vi "Read Configuration.vi"(10 "XML File Path conf":path=path "c:/ni-rt/startup/configuration.xml", 11 "Error In":errorcluster) -> (0 "Matrices":T1, 1 "Configuration":T3={"Accelerometer Bias"={"X (m/s)"=0.0, "Y (m/s)"=0.0, "Z (m/s)"=0.0}, "Gyroscope Bias"={"X (m/s)"=0.0, "Y (m/s)"=0.0, "Z (m/s)"=0.0}, "Steering Motor Gear Ratio"=611.0, "Steering Pully Gear Ratio"=1.0, "Steering Encoder CPR"=500.0, "Steering Motor Max RPM"=4000.0, "Wheelbase (m)"=1.12, "Fork Angle (rad)"=1.3, "Balancing Controller"={"Kp (/s)"=0.0, "Kd (1)"=0.0}, "Max Allowed Steering Angle (rad)"=0.7, "Task Periods"={"Emergency Stop (us)"=0, "IMU (us)"=0, "Steering Motor Encoder (us)"=0, "State Estimator (us)"=0, "Balancing Controller (us)"=0, "GNSS (us)"=0, "Logging (us)"=0, "Drive Motor (us)"=0}, "Drive Motor Gear Ratio"=0.7, "Drive Motor UART Delay (ms)"=10}, 3 "Error Out":errorcluster)   [LabVIEW 2021]
uses:
  Configuration.ctl
  <vilib>/Analysis/Matrix/Datatypes/RealMatrix.ctl
  <vilib>/Utility/xml.llb/Read From XML File(string).vi
  <vilib>/Analysis/Matrix/Numeric/Conversions/Matrix To Array - RM.vi
  <vilib>/Analysis/Matrix/NI_Matrix.lvlib
panel:
  in  "init trajectory":dbl[][](array[numeric])
  in  "XML File Path traj":path=path "c:/ni-rt/startup/trajectorylab.xml"
  in  "Init Matrix":T2
  in  "XML File Path matr":path=path "c:/ni-rt/startup/matrixlab.xml"
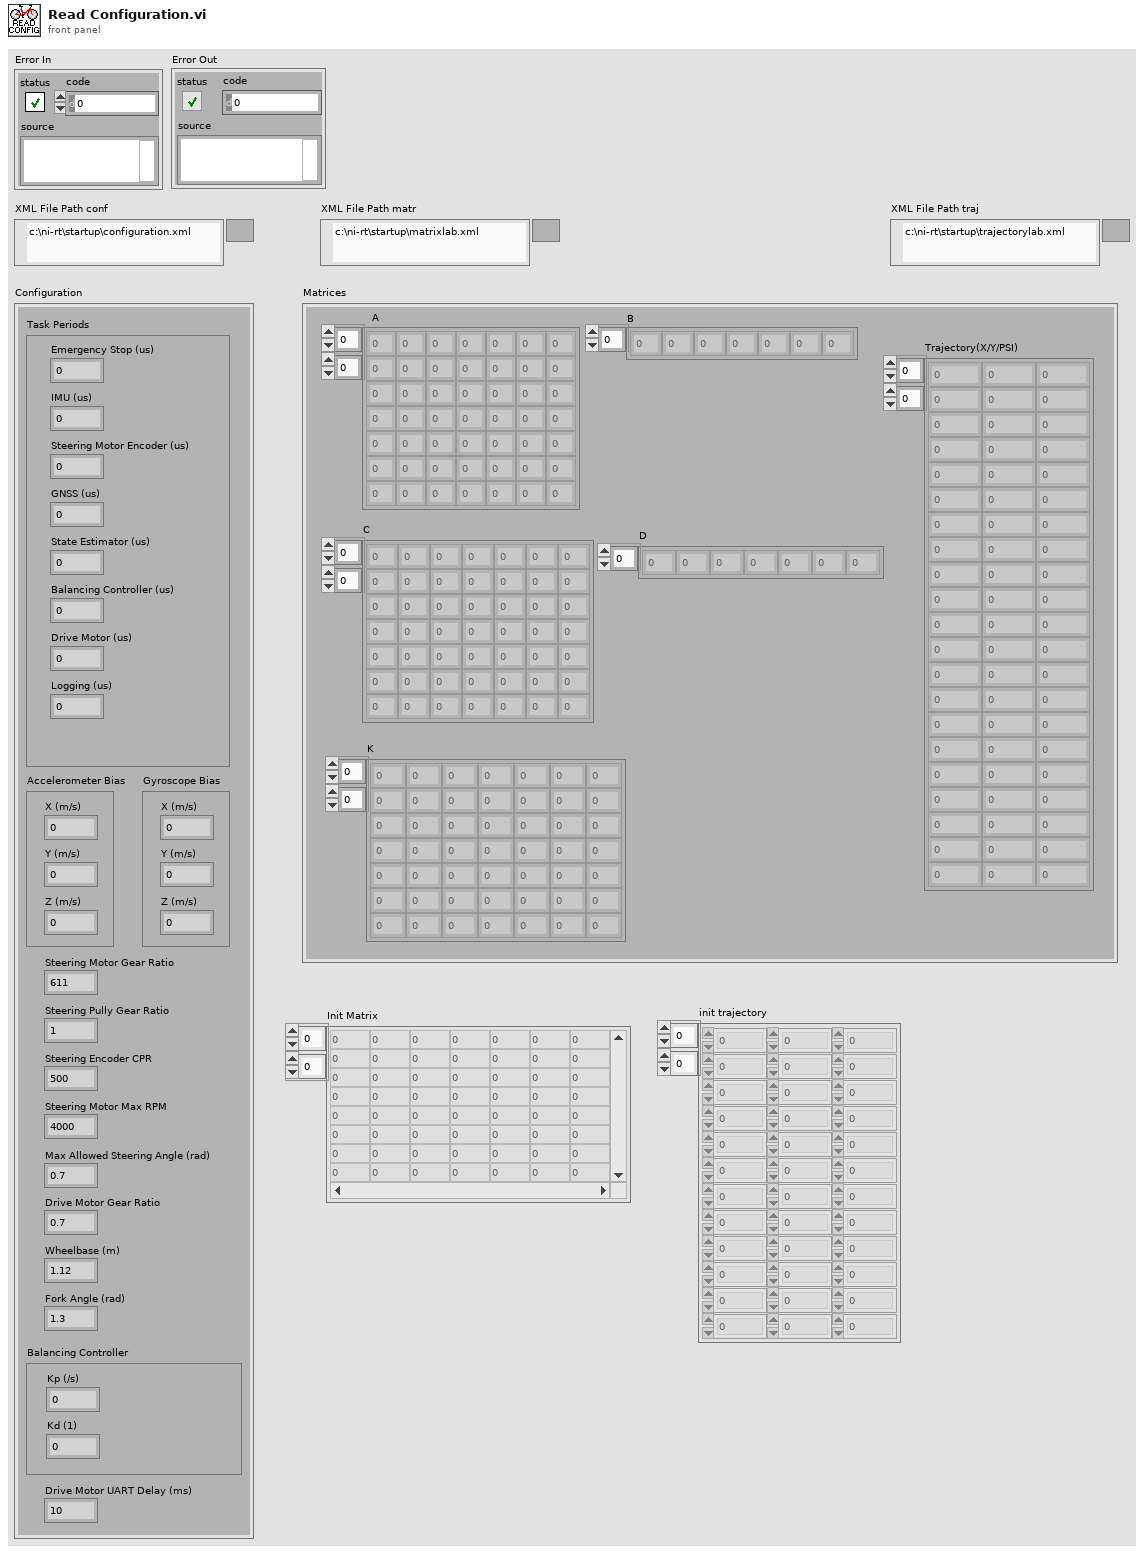
[diagram p1: front panel]
types:
  T1 = cluster{"B":dbl[], "A":dbl[][], "C":dbl[][], "D":dbl[], "K":dbl[][], "Trajectory(X/Y/PSI)":dbl[][]}
  T2 = typedef "NI_Matrix.lvlib/RealMatrix.ctl" = dbl[][]
  T3 = typedef "Configuration.ctl" = cluster{"Accelerometer Bias":cluster{"X (m/s)":dbl, "Y (m/s)":dbl, "Z (m/s)":dbl}, "Gyroscope Bias":cluster{"X (m/s)":dbl, "Y (m/s)":dbl, "Z (m/s)":dbl}, "Steering Motor Gear Ratio":dbl, "Steering Pully Gear Ratio":dbl, "Steering Encoder CPR":dbl, "Steering Motor Max RPM":dbl, "Wheelbase (m)":dbl, "Fork Angle (rad)":dbl, "Balancing Controller":cluster{"Kp (/s)":dbl, "Kd (1)":dbl}, "Max Allowed Steering Angle (rad)":dbl, "Task Periods":cluster{"Emergency Stop (us)":i64, "IMU (us)":i64, "Steering Motor Encoder (us)":i64, "State Estimator (us)":i64, "Balancing Controller (us)":i64, "GNSS (us)":i64, "Logging (us)":i64, "Drive Motor (us)":i64}, "Drive Motor Gear Ratio":dbl, "Drive Motor UART Delay (ms)":i64}
  T4 = cluster{"B":dbl[], "A":dbl[][], "C":dbl[][], "D":dbl[], "K":dbl[][], "Trajectory":dbl[][]}
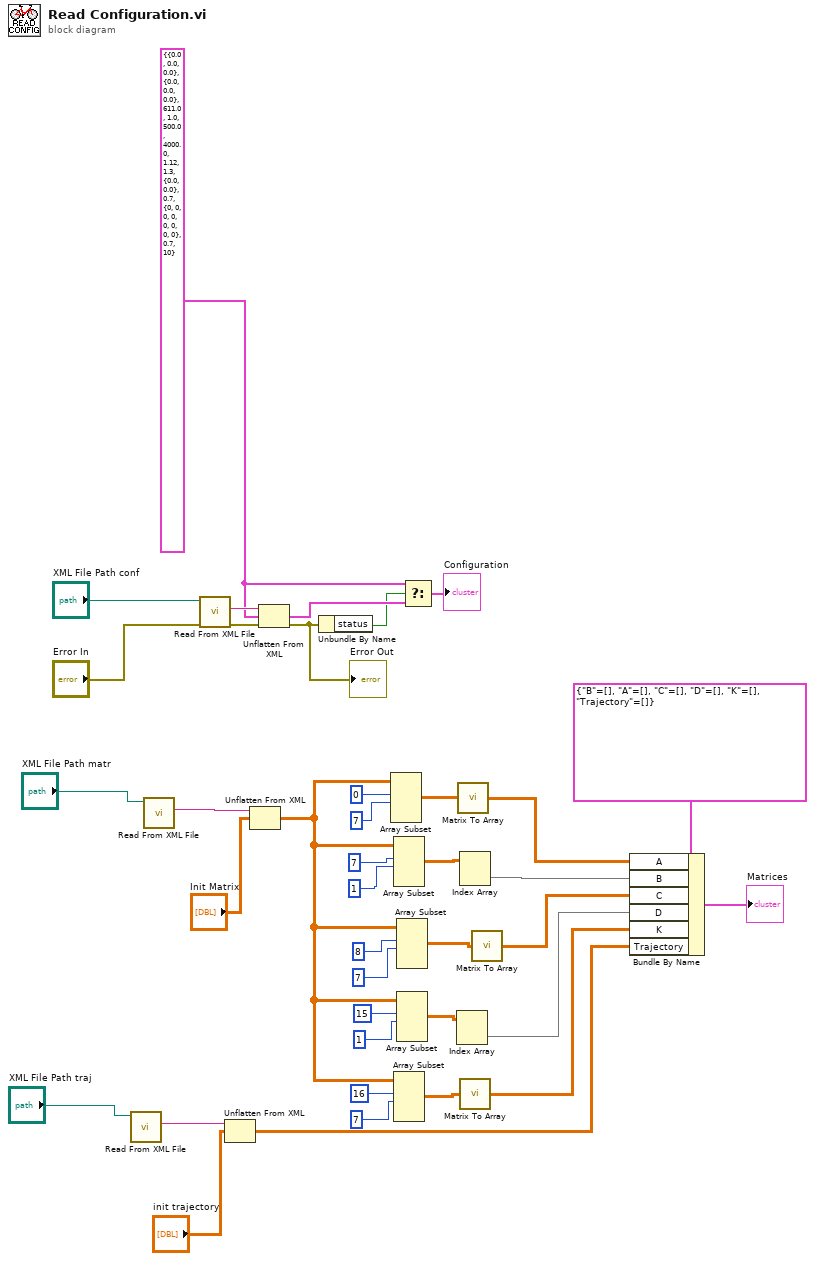
[diagram p0: block diagram]
diagram:
  w34 = T3 {"Accelerometer Bias"={"X (m/s)"=0.0, "Y (m/s)"=0.0, "Z (m/s)"=0.0}, "Gyroscope Bias"={"X (m/s)"=0.0, "Y (m/s)"=0.0, "Z (m/s)"=0.0}, "Steering Motor Gear Ratio"=611.0, "Steering Pully Gear Ratio"=1.0, "Steering Encoder CPR"=500.0, "Steering Motor Max RPM"=4000.0, "Wheelbase (m)"=1.12, "Fork Angle (rad)"=1.3, "Balancing Controller"={"Kp (/s)"=0.0, "Kd (1)"=0.0}, "Max Allowed Steering Angle (rad)"=0.7, "Task Periods"={"Emergency Stop (us)"=0, "IMU (us)"=0, "Steering Motor Encoder (us)"=0, "State Estimator (us)"=0, "Balancing Controller (us)"=0, "GNSS (us)"=0, "Logging (us)"=0, "Drive Motor (us)"=0}, "Drive Motor Gear Ratio"=0.7, "Drive Motor UART Delay (ms)"=10} ("Configuration")
  n1 = call-poly <vilib>:"Read From XML File.vi"("XML File Path"="XML File Path traj") -> ("XML Elements"=w3:string)  [unwired: 8 in, 2 out]
  n2 = call-poly <vilib>:"Read From XML File.vi"("XML File Path"="XML File Path matr") -> ("XML Elements"=w30:string)  [unwired: 8 in, 2 out]
  n3 = call-poly <vilib>:"Read From XML File.vi"("error in (no error)"="Error In", "XML File Path"="XML File Path conf") -> ("error out"=w39:errorcluster, "XML Elements"=w38:string)  [unwired: 7 in, 1 out]
  n4 = Unflatten From XML(xml string=w3, type="init trajectory") -> (value=w1:dbl[][])  [unwired: 1 in, 1 out]
  n5 = Unflatten From XML(xml string=w30, type="Init Matrix") -> (value=w13:T2)  [unwired: 1 in, 1 out]
  n6 = Unflatten From XML(xml string=w38, type=w34, error in (no error)=w39) -> (value=w33:T3, error out=w35:errorcluster)
  "Error Out" <- w35
  n7 = Unbundle By Name(w35) -> ("status"=w29:bool)
  n8 = Array Subset(array=w13, index (row)=0, length (row)=7) -> (w25:T2)  [unwired: 2 in]
  n9 = Array Subset(array=w13, index (row)=7, length (row)=1) -> (w10:T2)  [unwired: 2 in]
  n10 = Array Subset(array=w13, index (row)=16, length (row)=7) -> (w12:T2)  [unwired: 2 in]
  n11 = Array Subset(array=w13, index (row)=8, length (row)=7) -> (w17:T2)  [unwired: 2 in]
  n12 = Array Subset(array=w13, index (row)=15, length (row)=1) -> (w6:T2)  [unwired: 2 in]
  n13 = Select(t=w34, s=w29, f=w33) -> (s? t:f=→"Configuration":T3)
  n14 = Index Array(array=w6) -> (element=w5:dbl[])  [unwired: 2 in]
  n15 = call-poly <vilib>:"Matrix To Array.vi"("Real Matrix"=w25) -> ("Real 2D Array"=w22:dbl[][])
  n16 = Index Array(array=w10) -> (element=w7:dbl[])  [unwired: 2 in]
  n17 = call-poly <vilib>:"Matrix To Array.vi"("Real Matrix"=w12) -> ("Real 2D Array"=w11:dbl[][])
  n18 = call-poly <vilib>:"Matrix To Array.vi"("Real Matrix"=w17) -> ("Real 2D Array"=w16:dbl[][])
  n19 = Bundle By Name(cluster=T4 {"B"=[], "A"=[], "C"=[], "D"=[], "K"=[], "Trajectory"=[]}, "A"=w22, "B"=w7, "C"=w16, "D"=w5, "K"=w11, "Trajectory"=w1) -> (→"Matrices":T4)
